vi "Stop Core.vi"(10 "final error code":i32, 11 "SensorView in":refnum<class "SensorView.lvclass">) -> (3 "SensorView out":refnum<class "SensorView.lvclass">)   [LabVIEW 2012, in "Sensor Definition.lvlib" / "SensorView.lvclass"]
doc: "(<B>Filename</B>: Actor Framework.lvlib:Actor.lvclass:Stop Core.vi)\n\nDefines what the actor does before it stops. Use the <B>final error code</B> input to determine whether the actor shut down in response to an error.\n\nBy default, this method does nothing. A descendant class may override it to define behavior, such as shutting down any processes the actor initiated in its override of the Actor Core method."
uses:
  SensorView.lvclass
  <vilib>/ActorFramework/Actor/Actor.lvclass/Actor.ctl
  <vilib>/ActorFramework/Message Enqueuer/Message Enqueuer.lvclass/Message Enqueuer.ctl
  SensorView.lvclass/SensorView.ctl
  Win8uiFramework/ViewableActor.lvclass
  Sensor Messages/Unsubscribe SensorView Msg/Unsubscribe SensorView Msg.lvclass/Unsubscribe SensorView Msg.ctl
  Read SensorInfo Changed Event.vi
  Read SensorData Changed Event.vi
  <vilib>/ActorFramework/Message Enqueuer/Init from Existing Queue.vi
  <vilib>/ActorFramework/Message Enqueuer/Enqueue.vi
  <vilib>/ActorFramework/Message Priority Queue/Priority Enqueue.vi
  <vilib>/ActorFramework/Message Enqueuer/Message Enqueuer.lvclass
  SensorData.lvclass
  Sensor Messages/Unsubscribe SensorView Msg/Unsubscribe SensorView Msg.lvclass
  <vilib>/ActorFramework/Actor/Actor.lvclass
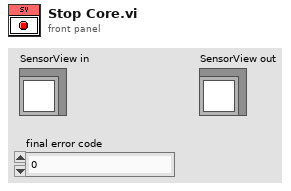
[diagram p1: front panel]
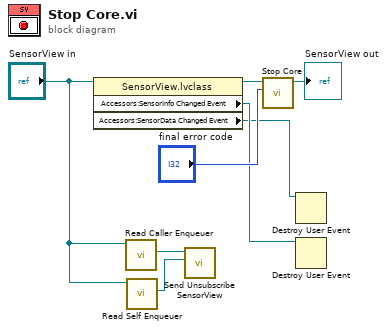
[diagram p0: block diagram]
diagram:
  n1 = property class="SensorView.lvclass"(reference="SensorView in") -> (reference out=w6:refnum<class "SensorView.lvclass">, "Accessors:SensorInfo Changed Event"=w5:refnum<user-event>, "Accessors:SensorData Changed Event"=w4:refnum<user-event>)  [unwired: 1 in, 1 out]
  n2 = call <vilib>:"Read Caller Enqueuer.vi"("Actor"="SensorView in") -> ("Caller Enqueuer"=w3:refnum<class "Message Enqueuer.lvclass">)  [unwired: 10 in]
  n3 = call <vilib>:"Read Self Enqueuer.vi"("Actor"="SensorView in") -> ("Self Enqueuer"=w1:refnum<class "Message Enqueuer.lvclass">)  [unwired: 10 in]
  n4 = call "Send Unsubscribe SensorView.vi"("SensorView Enqueuer"=w1, "Message Enqueuer"=w3) -> ()  [unwired: 8 in, 2 out]
  n5 = call-parent "Stop Core.vi"("final error code"="final error code", "ViewableActor in"=w6) -> ("ViewableActor out"=→"SensorView out":refnum<class "SensorView.lvclass">)  [unwired: 9 in]
  n6 = Destroy User Event(user event=w4) -> ()  [unwired: 1 in, 1 out]
  n7 = Destroy User Event(user event=w5) -> ()  [unwired: 1 in, 1 out]
